vi "SetRedLevel.vi"(0 "error in":errorcluster, 2 "Red Light Level":sgl, 3 "node":string) -> (1 "error out":errorcluster)   [LabVIEW 2012]
doc: "Sets the red light on Baxter's head to a given level"
uses:
  <userlib>/ROSforLV/ROS/Code/Console/Servers/ServerSubs/TopicDef.ctl
  <userlib>/ROSforLV/ROS/Code/SubVIs/_ROSDirection.ctl
  <userlib>/ROSforLV/ROS/MessageBuilding/std_msgs/subs/float32Scalar.vi
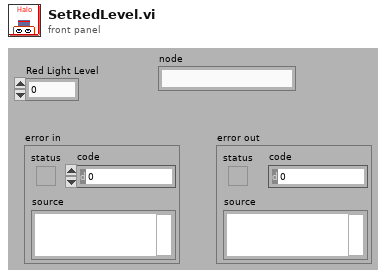
[diagram p1: front panel]
types:
  T1 = typedef "TopicDef.ctl" = cluster{"Topic":string, "Type":string, "Action":T2, "Update (ms)":u16, "queue size":u16}
  T2 = typedef "_ROSDirection.ctl" = enum16{"Node", "Publisher", "Subscriber", "ServiceClient", "ServiceProvider"}
  T3 = typedef "_ROSControl.ctl" = cluster{"topic port":u16, "Node":string, "topic":string, "type":string, "node port":u16, "error ":errorcluster, "Direction":T2, "Update (ms)":u16, "FIFO size":u16}
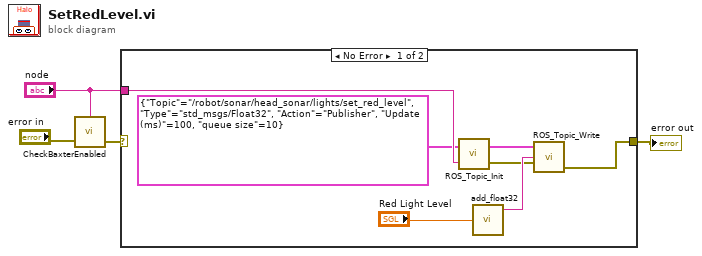
[diagram p0: block diagram]
diagram:
  n1 = call <userlib>:"CheckBaxterEnabled.vi"("error in"="error in", "node"="node") -> ("error out"=w2:errorcluster)  [unwired: 2 in]
  n2 = case shown="No Error" w2 {
    selector: w2 -> [_ w12]
    tunnel: [w5 w12] -> w4
    tunnel: "node" -> [w10 _]
    frame No Error {
      n3 = call <userlib>:"ROS_Topic_Init.vi"("node"=w10, "Definitions"=T1 {"Topic"="/robot/sonar/head_sonar/lights/set_red_level", "Type"="std_msgs/Float32", "Action"=enum."Publisher", "Update (ms)"=100, "queue size"=10}) -> ("error out"=w6:errorcluster, "ROS out"=w11:T3)
      n4 = call-poly <userlib>:"add_float32.vi"("Numeric"="Red Light Level") -> ("msg out"=w7:string)  [unwired: 4 in]
      n5 = call <userlib>:"ROS_Topic_Write.vi"("error in (no error)"=w6, "Msg in"=w7, "ROS in"=w11) -> ("error out"=w5:errorcluster)  [unwired: 1 in, 1 out]
    }
    frame Error {
    }
  }
  "error out" <- w4
